vi "Carriage Intake Immediate with Deadband.vi"(4 "Grab":bool, 6 "Extend":bool, 7 "Description":string, 8 "Command Info In":T1, 9 "Deadband Value":dbl=0.01, 11 "Setpoint":dbl) -> (0 "Command Info Out":T1)   [LabVIEW 2018]
doc: "This template includes code for deadband comparision to avoid excessive command scheduling. It is particularly useful for joystick-driven commands.\n\nBe sure to right-click and select New from Template and save with a new command name."
uses:
  <vilib>/Rock Robotics/WPI/Framework/Command Status Info.ctl
  <vilib>/Rock Robotics/WPI/Framework/Completion Status.ctl
  <vilib>/Rock Robotics/WPI/Framework/Completion Notifier.ctl
  Implementation/Carriage Intake Setpoints.ctl
  Implementation/Carriage Intake Operations.ctl
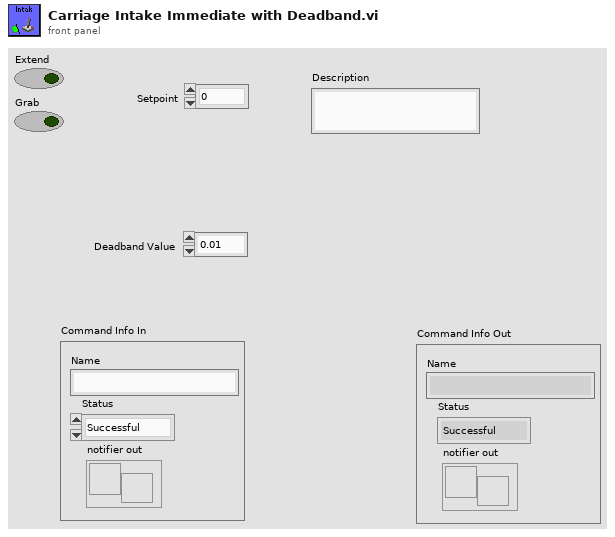
[diagram p1: front panel]
types:
  T1 = typedef "Command Status Info.ctl" = cluster{"Name":string, "Status":T2, "notifier out":T3}
  T2 = typedef "Completion Status.ctl" = enum16{"Successful", "Aborted", "Incomplete"}
  T3 = typedef "Completion Notifier.ctl" = refnum<notifier>
  T4 = typedef "Carriage Intake Setpoints.ctl" = cluster{"Operation":T5, "Setpoint":dbl, "Duration":dbl, "Extend":bool, "Grab":bool}
  T5 = typedef "Carriage Intake Operations.ctl" = enum16{"Reserve", "Read Current", "Immediate"}
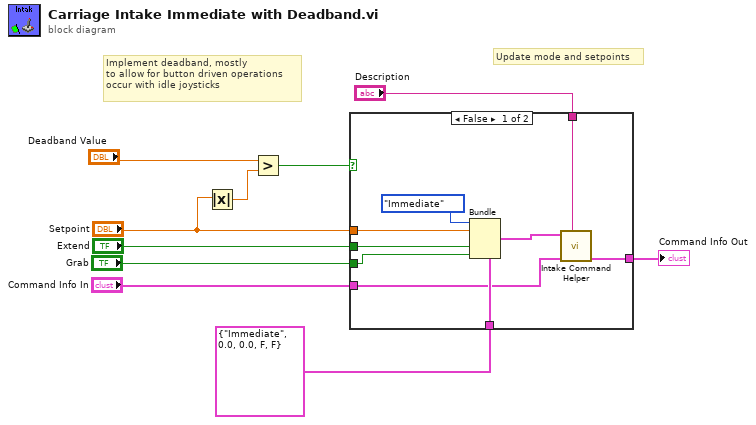
[diagram p0: block diagram]
diagram:
  # "Implement deadband, mostly\nto allow for button driven operations\noccur with idle joysticks"
  # "Update mode and setpoints"
  n1 = Absolute Value(x="Setpoint") -> (abs(x)=w9:dbl)
  n2 = Greater?(x="Deadband Value", y=w9) -> (0:w3:bool)
  n3 = case shown="False" w3 {
    tunnel: "Setpoint" -> [w19 _]
    tunnel: T4 {"Operation"=enum."Immediate", "Setpoint"=0.0, "Duration"=0.0, "Extend"=FALSE, "Grab"=FALSE} ("SubSystem Data") -> [w18 _]
    tunnel: [w17 w20] -> w8
    tunnel: "Command Info In" -> [w16 w20]
    tunnel: "Description" -> [w14 _]
    tunnel: "Extend" -> [w13 _]
    tunnel: "Grab" -> [w11 _]
    frame False {
      n4 = Bundle(cluster=w18, "Operation"=Carriage_Intake_Operations."Immediate", "Setpoint"=w19, "Extend"=w13, "Grab"=w11) -> (w15:T4)  [unwired: 1 in]
      n5 = call "Intake Command Helper.vi"("Description"=w14, "Command Info In"=w16, "SubSystem Data"=w15) -> ("Command Info Out"=w17:T1)  [unwired: 6 in, 2 out]
    }
    frame True {
    }
  }
  "Command Info Out" <- w8
